vi "DeleteBlank.vi"(10 "Transmit":string[][](table)=[["33C", "0", "8", "02", "00", "00", "00", "00", "00", "00", "00", "100"], ["35C", "0", "8", "14", "00", "A9", "80", "4A", "94", "A0", "09", "100"], ["395", "0", "8", "00", "00", "00", "00", "00", "00", "00", "00", "100"], ["581", "0", "8", "81", "00", "00", "00", "00", "00", "00", "00", "500"], ["38F", "0", "8", "00", "00", "00", "00", "00", "00", "00", "00", "100"], ["", "", "", "", "", "", "", "", "", "", "", ""]]) -> (2 "Transmit out":string[][](array[string]))   [LabVIEW 2020]
panel:
  out "大小 2":i32[](array[numeric])
  out "大小":i32[](array[numeric])
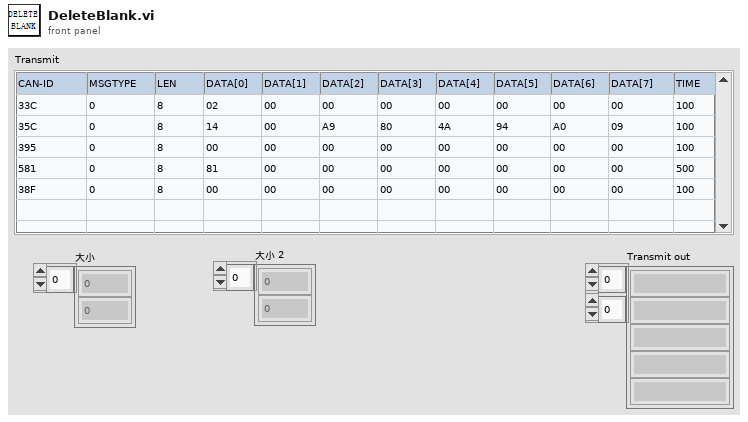
[diagram p1: front panel]
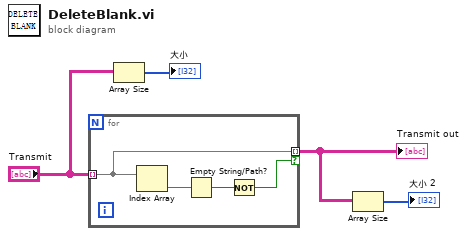
[diagram p0: block diagram]
diagram:
  n1 = for {
    tunnel: "Transmit" -> [w7] mode=indexing
    tunnel: [w7] -> w1 mode=indexing if=w5
    n2 = Index Array(array=w7) -> (element=w8:string)  [unwired: 1 in]
    n3 = Empty String/Path?(string/path=w8) -> (empty?=w6:bool)
    n4 = Not(x=w6) -> (.not. x?=w5:bool)
  }
  "Transmit out" <- w1
  n5 = Array Size(array="Transmit") -> (size(s)=→"大小":i32[])
  n6 = Array Size(array=w1) -> (size(s)=→"大小 2":i32[])
